vi "ROI group-Tick group ROIs show_hide option.vi"(8 "error in (no error)":errorcluster, 10 "Valid?":bool, 11 "Menu in":refnum<k9>) -> (0 "error out":errorcluster, 3 "Menu out":refnum<k9>)   [LabVIEW 2013]
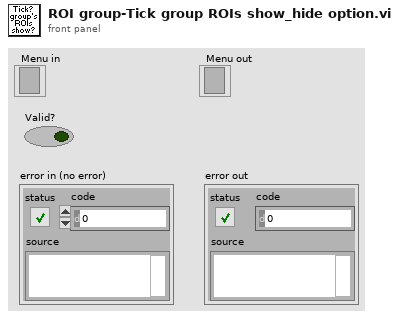
[diagram p1: front panel]
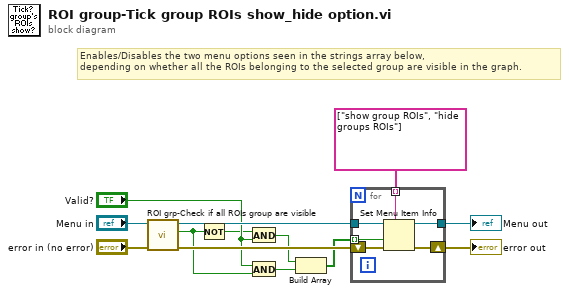
[diagram p0: block diagram]
diagram:
  # "Enables/Disables the two menu options seen in the strings array below,\ndepending on whether all the ROIs belonging to the selected group are visible in the graph."
  n1 = call "ROI grp-Check if all ROIs group are visible.vi"("error in (no error)"="error in (no error)") -> ("error out"=w9:errorcluster, "Group's ROIs are all visible"=w6:bool)  [unwired: 9 in]
  n2 = Not(x=w6) -> (.not. x?=w1:bool)
  n3 = And(x=w1, y="Valid?") -> (x .and. y?=w3:bool)
  n4 = And(x="Valid?", y=w6) -> (x .and. y?=w4:bool)
  n5 = Build Array(w3, w4) -> (w2:bool[])
  n6 = for {
    tunnel: "Menu in" -> [w18]
    tunnel: string[] ["show group ROIs", "hide groups ROIs"] -> [w17] mode=indexing
    tunnel: w2 -> [w14] mode=indexing
    shift-right: [w15] -> w10
    shift-left: w9 -> [w16]
    tunnel: [w13] -> w12
    n7 = Set Menu Item Info(7:w17, 8:w16, 9:w14, 11:w18) -> (0:w15:errorcluster, 3:w13:refnum<k9>)  [unwired: 3 in]
  }
  "error out" <- w10
  "Menu out" <- w12
